vi "运行时间输出.vi"(11 "初始化":bool) -> (2 "Elapsed Time (s)":dbl, 3 "Time has Elapsed":bool)   [LabVIEW 2016, in "斯坦道多参数.lvlib"]
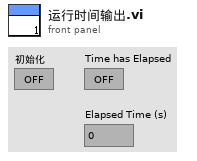
[diagram p1: front panel]
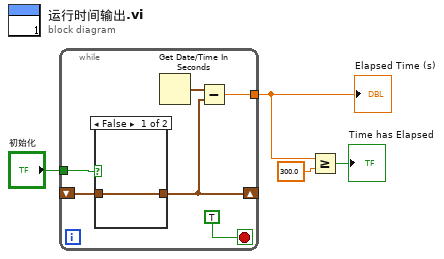
[diagram p0: block diagram]
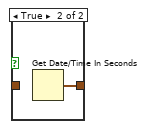
[diagram p2: hidden frame]
diagram:
  n1 = while {
    tunnel: "初始化" -> [w10]
    shift-right: [w7] -> _
    shift-left: _ -> [w9]
    tunnel: [w5] -> w3
    stop <- TRUE stop-if-true
    n2 = case shown="False" w10 {
      tunnel: [w11 w12] -> w7
      tunnel: w9 -> [w11 _]
      frame False {
      }
      frame True {
        n3 = Get Date/Time In Seconds() -> (seconds since 1Jan1904=w12:timestamp)
      }
    }
    n4 = Get Date/Time In Seconds() -> (seconds since 1Jan1904=w8:timestamp)
    n5 = Subtract(x=w8, y=w7) -> (x-y=w5:dbl)
  }
  "Elapsed Time (s)" <- w3
  n6 = Greater Or Equal?(x=w3, y=300.0) -> (x >= y?=→"Time has Elapsed":bool)
